vi "SessionCfgLoad.vi"(8 "error in (no error)":errorcluster, 11 "This VI":refnum<vi>) -> (0 "error out":errorcluster)   [LabVIEW 2019]
uses:
  <vilib>/Utility/config.llb/Read Key (String).vi
  <vilib>/Utility/config.llb/NI_LVConfig.lvlib
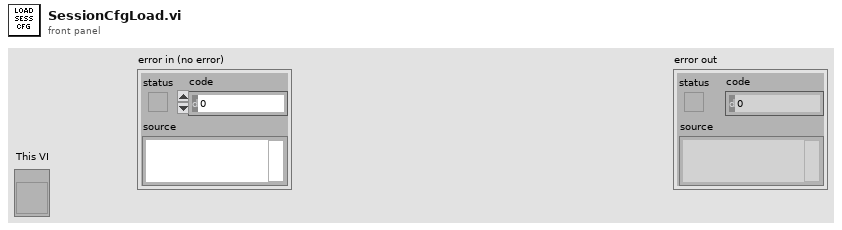
[diagram p1: front panel]
types:
  T1 = typedef "NI_LVConfig.lvlib/Config Data RefNum.ctl" = refnum<k1>
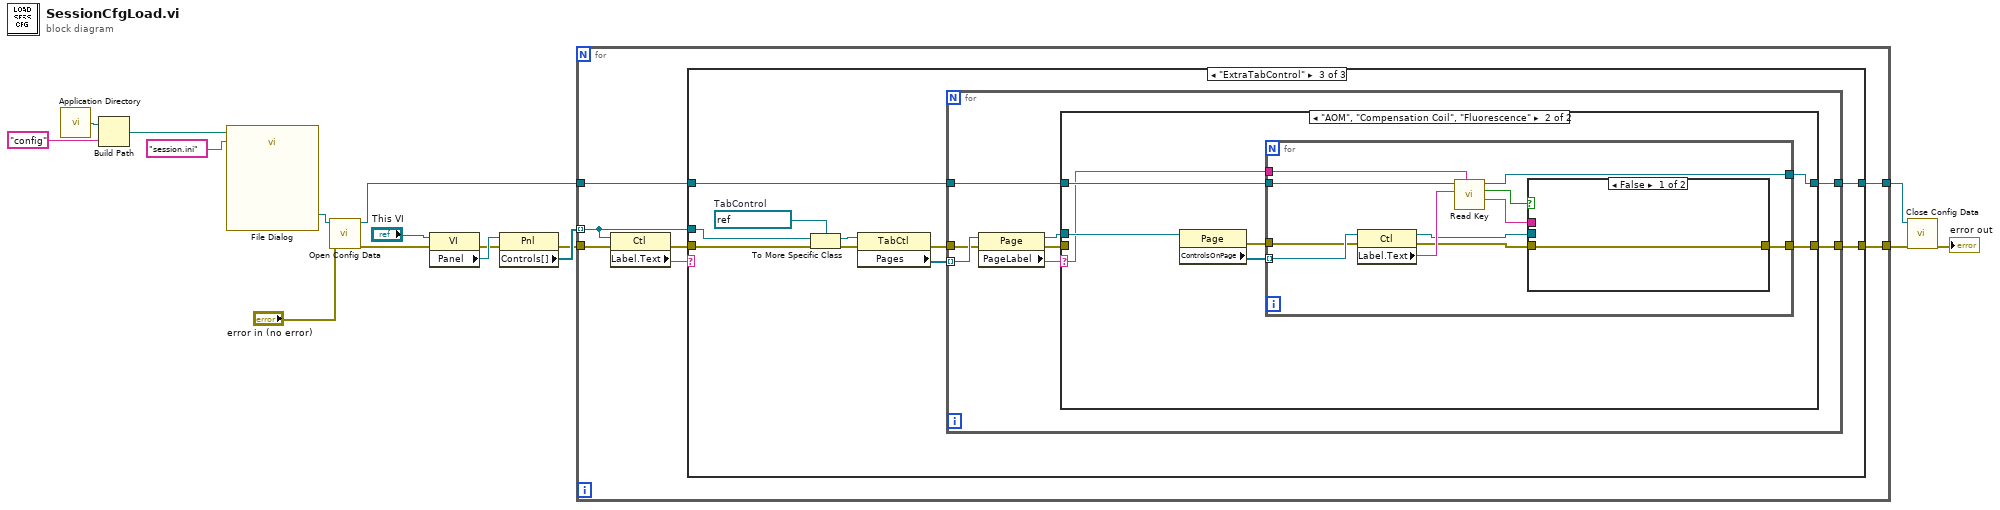
[diagram p0: block diagram]
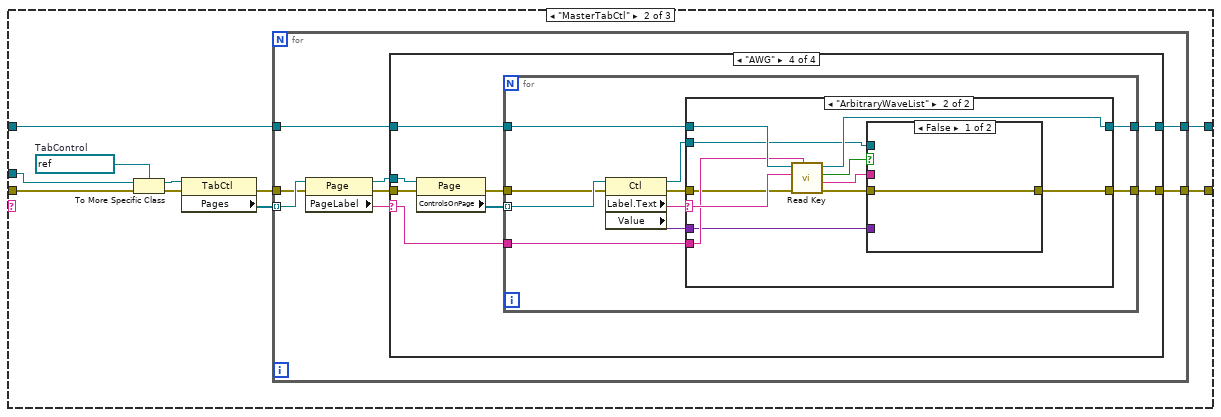
[diagram p3: hidden frame]
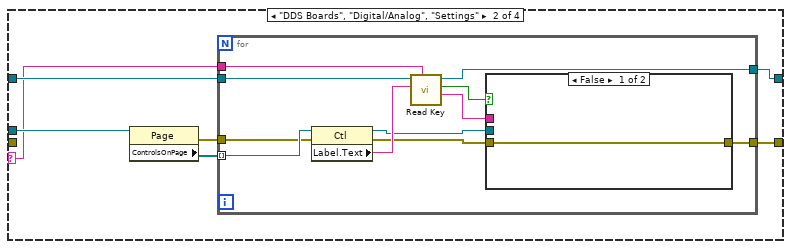
[diagram p5: hidden frame]
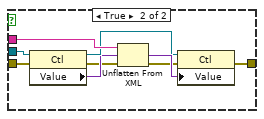
[diagram p6: hidden frame]
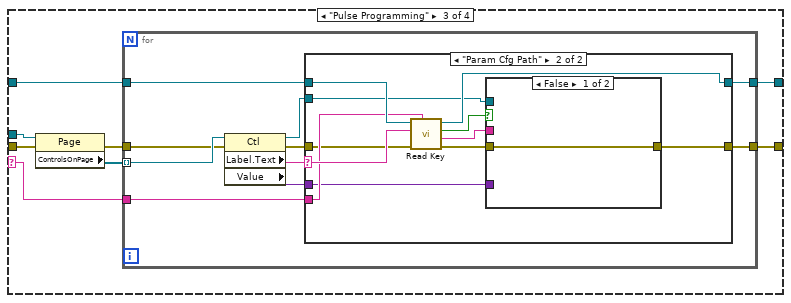
[diagram p7: hidden frame]
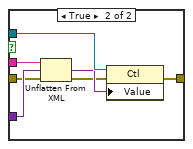
[diagram p9: hidden frame]
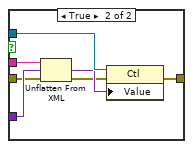
[diagram p11: hidden frame]
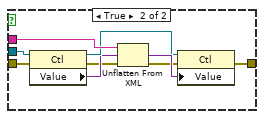
[diagram p13: hidden frame]
diagram:
  n1 = call <vilib>:"Application Directory.vi"() -> ("Application Directory"=w9:path)
  n2 = Build Path(base path=w9, name or relative path="config") -> (appended path=w8:path)
  n3 = call "File Dialog"("start path"=w8, "default name"="session.ini") -> ("selected path"=w11:path)  [unwired: 10 in, 3 out]
  n4 = call <vilib>:"Open Config Data.vi"("error in (no error)"="error in (no error)", "configuration file path"=w11) -> ("error out"=w6:errorcluster, "refnum"=w13:T1)  [unwired: 7 in, 1 out]
  n5 = property class="VI"(reference="This VI", error in=w6) -> (error out=w15:errorcluster, "Panel"=w16:refnum<vi>)  [unwired: 1 out]
  n6 = property class="Pnl"(reference=w16, error in=w15) -> (error out=w5:errorcluster, "Controls[]"=w14:refnum<vi>[])  [unwired: 1 out]
  n7 = for {
    tunnel: w14 -> [w23] mode=indexing
    tunnel: w13 -> [w21]
    tunnel: [w20] -> w12
    tunnel: w5 -> [w19]
    tunnel: [w17] -> w4
    n8 = property class="Ctl"(reference=w23, error in=w19) -> (error out=w18:errorcluster, "Label.Text"=w22:string)  [unwired: 1 out]
    n9 = case shown="\"ExtraTabControl\"" w22 {
      tunnel: w23 -> [_ w32 w158]
      tunnel: w21 -> [w25 w31 w157]
      tunnel: [w25 w30 w156] -> w20
      tunnel: w18 -> [w24 w29 w155]
      tunnel: [w24 w26 w152] -> w17
      frame "False", Default {
      }
      frame "MasterTabCtl" {
        w35 = refnum<vi> refnum  # TabControl
        n10 = To More Specific Class(target class=w35, reference=w32, error in=w29) -> (specific class reference=w34:refnum<vi>, error out=w28:errorcluster)
        n11 = property class="TabCtl"(reference=w34, error in=w28) -> (error out=w27:errorcluster, "Pages"=w33:refnum<vi>[])  [unwired: 1 out]
        n12 = for {
          tunnel: w33 -> [w43] mode=indexing
          tunnel: w31 -> [w40]
          tunnel: [w39] -> w30
          tunnel: w27 -> [w38]
          tunnel: [w36] -> w26
          n13 = property class="Page"(reference=w43, error in=w38) -> (reference out=w41:refnum<vi>, error out=w37:errorcluster, "PageLabel"=w42:string)
          n14 = case shown="\"AWG\"" w42 {
            selector: w42 -> [_ w49 w79 w118]
            tunnel: w41 -> [_ w52 w80 w119]
            tunnel: w40 -> [w45 w50 w78 w117]
            tunnel: [w45 w48 w77 w116] -> w39
            tunnel: w37 -> [w44 _ w76 w115]
            tunnel: [w44 w46 w74 w113] -> w36
            frame "False", Default {
            }
            frame "DDS Boards", "Digital/Analog", "Settings" {
              n15 = property class="Page"(reference=w52) -> (error out=w47:errorcluster, "ControlsOnPage"=w51:refnum<vi>[])  [unwired: 1 in, 1 out]
              n16 = for {
                tunnel: w51 -> [w63] mode=indexing
                tunnel: w50 -> [w60]
                tunnel: w49 -> [w61]
                tunnel: [w59] -> w48
                tunnel: w47 -> [w55]
                tunnel: [w53] -> w46
                n17 = property class="Ctl"(reference=w63, error in=w55) -> (reference out=w56:refnum<vi>, error out=w54:errorcluster, "Label.Text"=w62:string)
                n18 = call-poly <vilib>:"Read Key.vi"("section"=w61, "key"=w62, "refnum"=w60) -> ("value"=w57:string, "found?"=w58:bool, "refnum out"=w59:T1)  [unwired: 5 in, 1 out]
                n19 = case shown="False" w58 {
                  tunnel: w57 -> [_ w72]
                  tunnel: w56 -> [_ w71]
                  tunnel: w54 -> [w64 w68]
                  tunnel: [w64 w65] -> w53
                  frame False {
                  }
                  frame True {
                    n20 = property class="Ctl"(reference=w71, error in=w68) -> (reference out=w70:refnum<vi>, error out=w67:errorcluster, "Value"=w69:variant)
                    n21 = Unflatten From XML(xml string=w72, type=w69, error in (no error)=w67) -> (value=w73:variant, error out=w66:errorcluster)
                    n22 = property class="Ctl"(reference=w70, error in=w66, "Value"=w73) -> (error out=w65:errorcluster)  [unwired: 1 out]
                  }
                }
              }
            }
            frame "Pulse Programming" {
              n23 = property class="Page"(reference=w80, error in=w76) -> (error out=w75:errorcluster, "ControlsOnPage"=w81:refnum<vi>[])  [unwired: 1 out]
              n24 = for {
                tunnel: w81 -> [w91] mode=indexing
                tunnel: w78 -> [w88]
                tunnel: [w87] -> w77
                tunnel: w79 -> [w86]
                tunnel: w75 -> [w84]
                tunnel: [w82] -> w74
                n25 = property class="Ctl"(reference=w91, error in=w84) -> (reference out=w85:refnum<vi>, error out=w83:errorcluster, "Label.Text"=w90:string, "Value"=w89:variant)
                n26 = case shown="\"Param Cfg Path\"" w90 {
                  selector: w90 -> [_ w102]
                  tunnel: w89 -> [_ w100]
                  tunnel: w88 -> [w93 w104]
                  tunnel: [w93 w103] -> w87
                  tunnel: w86 -> [_ w101]
                  tunnel: w85 -> [_ w97]
                  tunnel: w83 -> [w92 w96]
                  tunnel: [w92 w94] -> w82
                  frame "False", Default {
                  }
                  frame "Param Cfg Path" {
                    n27 = call-poly <vilib>:"Read Key.vi"("section"=w101, "error in (no error)"=w96, "key"=w102, "refnum"=w104) -> ("error out"=w95:errorcluster, "value"=w98:string, "found?"=w99:bool, "refnum out"=w103:T1)  [unwired: 4 in]
                    n28 = case shown="False" w99 {
                      tunnel: w100 -> [_ w112]
                      tunnel: w98 -> [_ w111]
                      tunnel: w97 -> [_ w110]
                      tunnel: w95 -> [w105 w108]
                      tunnel: [w105 w106] -> w94
                      frame False {
                      }
                      frame True {
                        n29 = Unflatten From XML(xml string=w111, type=w112, error in (no error)=w108) -> (value=w109:variant, error out=w107:errorcluster)
                        n30 = property class="Ctl"(reference=w110, error in=w107, "Value"=w109) -> (error out=w106:errorcluster)  [unwired: 1 out]
                      }
                    }
                  }
                }
              }
            }
            frame "AWG" {
              n31 = property class="Page"(reference=w119, error in=w115) -> (error out=w114:errorcluster, "ControlsOnPage"=w120:refnum<vi>[])  [unwired: 1 out]
              n32 = for {
                tunnel: w120 -> [w130] mode=indexing
                tunnel: w117 -> [w127]
                tunnel: [w126] -> w116
                tunnel: w118 -> [w125]
                tunnel: w114 -> [w123]
                tunnel: [w121] -> w113
                n33 = property class="Ctl"(reference=w130, error in=w123) -> (reference out=w124:refnum<vi>, error out=w122:errorcluster, "Label.Text"=w129:string, "Value"=w128:variant)
                n34 = case shown="\"ArbitraryWaveList\"" w129 {
                  selector: w129 -> [_ w141]
                  tunnel: w128 -> [_ w139]
                  tunnel: w127 -> [w132 w143]
                  tunnel: [w132 w142] -> w126
                  tunnel: w125 -> [_ w140]
                  tunnel: w124 -> [_ w136]
                  tunnel: w122 -> [w131 w135]
                  tunnel: [w131 w133] -> w121
                  frame "False", Default {
                  }
                  frame "ArbitraryWaveList" {
                    n35 = call-poly <vilib>:"Read Key.vi"("section"=w140, "error in (no error)"=w135, "key"=w141, "refnum"=w143) -> ("error out"=w134:errorcluster, "value"=w137:string, "found?"=w138:bool, "refnum out"=w142:T1)  [unwired: 4 in]
                    n36 = case shown="False" w138 {
                      tunnel: w139 -> [_ w151]
                      tunnel: w137 -> [_ w150]
                      tunnel: w136 -> [_ w149]
                      tunnel: w134 -> [w144 w147]
                      tunnel: [w144 w145] -> w133
                      frame False {
                      }
                      frame True {
                        n37 = Unflatten From XML(xml string=w150, type=w151, error in (no error)=w147) -> (value=w148:variant, error out=w146:errorcluster)
                        n38 = property class="Ctl"(reference=w149, error in=w146, "Value"=w148) -> (error out=w145:errorcluster)  [unwired: 1 out]
                      }
                    }
                  }
                }
              }
            }
          }
        }
      }
      frame "ExtraTabControl" {
        w161 = refnum<vi> refnum  # TabControl
        n39 = To More Specific Class(target class=w161, reference=w158, error in=w155) -> (specific class reference=w160:refnum<vi>, error out=w154:errorcluster)
        n40 = property class="TabCtl"(reference=w160, error in=w154) -> (error out=w153:errorcluster, "Pages"=w159:refnum<vi>[])  [unwired: 1 out]
        n41 = for {
          tunnel: w159 -> [w169] mode=indexing
          tunnel: w157 -> [w166]
          tunnel: [w165] -> w156
          tunnel: w153 -> [w164]
          tunnel: [w162] -> w152
          n42 = property class="Page"(reference=w169, error in=w164) -> (reference out=w167:refnum<vi>, error out=w163:errorcluster, "PageLabel"=w168:string)
          n43 = case shown="\"AOM\", \"Compensation Coil\", \"Fluorescence\"" w168 {
            selector: w168 -> [_ w175]
            tunnel: w167 -> [_ w178]
            tunnel: w166 -> [w171 w176]
            tunnel: [w171 w174] -> w165
            tunnel: w163 -> [w170 _]
            tunnel: [w170 w172] -> w162
            frame "False", Default {
            }
            frame "AOM", "Compensation Coil", "Fluorescence" {
              n44 = property class="Page"(reference=w178) -> (error out=w173:errorcluster, "ControlsOnPage"=w177:refnum<vi>[])  [unwired: 1 in, 1 out]
              n45 = for {
                tunnel: w177 -> [w189] mode=indexing
                tunnel: w176 -> [w186]
                tunnel: w175 -> [w187]
                tunnel: [w185] -> w174
                tunnel: w173 -> [w181]
                tunnel: [w179] -> w172
                n46 = property class="Ctl"(reference=w189, error in=w181) -> (reference out=w182:refnum<vi>, error out=w180:errorcluster, "Label.Text"=w188:string)
                n47 = call-poly <vilib>:"Read Key.vi"("section"=w187, "key"=w188, "refnum"=w186) -> ("value"=w183:string, "found?"=w184:bool, "refnum out"=w185:T1)  [unwired: 5 in, 1 out]
                n48 = case shown="False" w184 {
                  tunnel: w183 -> [_ w198]
                  tunnel: w182 -> [_ w197]
                  tunnel: w180 -> [w190 w194]
                  tunnel: [w190 w191] -> w179
                  frame False {
                  }
                  frame True {
                    n49 = property class="Ctl"(reference=w197, error in=w194) -> (reference out=w196:refnum<vi>, error out=w193:errorcluster, "Value"=w195:variant)
                    n50 = Unflatten From XML(xml string=w198, type=w195, error in (no error)=w193) -> (value=w199:variant, error out=w192:errorcluster)
                    n51 = property class="Ctl"(reference=w196, error in=w192, "Value"=w199) -> (error out=w191:errorcluster)  [unwired: 1 out]
                  }
                }
              }
            }
          }
        }
      }
    }
  }
  n52 = call <vilib>:"Close Config Data.vi"("error in (no error)"=w4, "refnum"=w12) -> ("error out"=→"error out":errorcluster)  [unwired: 8 in, 1 out]
